vi "arch spiral FGV.vi"(0 "X Start":fxp<+/-,32,16>, 1 "Spiral Step Size":fxp<+/-,32,16>, 2 "Max radius":fxp<+/-,32,16>, 5 "Y Start":fxp<+/-,32,16>, 7 "Action":T1, 9 "Spiral Rotation Direction":T3, 11 "Radial direction":T2=enum."Inward", 12 "Det Frequency":fxp<+,32,0>=0.9999999997671694, 13 "Traj Frequency":fxp<+,32,0>=0.9999999997671694) -> (4 "X position":fxp<+/-,32,16>, 6 "Y position":fxp<+/-,32,16>, 10 "Number of positions":u32, 15 "Trajectory Complete":bool)   [LabVIEW 2015]
uses:
  spiral rotation direction.ctl
  spiral radial direction.ctl
  Trajectory FGV states.ctl
  <vilib>/rvi/FXPMathLib/FxpSinAndCos/subVIs/nifxpmath_SinAndCos_SimConfig.ctl
  <vilib>/rvi/Emulation/niFpgaGetClockAttributes.vi
  <vilib>/rvi/Emulation/niFpgaSctlEmulationGetInTimedLoop.vi
  <vilib>/rvi/Emulation/niFpgaEmulationReportErrorSimple.vi
  <vilib>/rvi/FXPMathLib/FxpSinAndCos/simVIs/DllFxpSinAndCosTemp_sub.vi
  <vilib>/rvi/Emulation/niFpgaCriticalErrorInLSC.vi
  <vilib>/rvi/FXPMathLib/FxpSinAndCos/XNode/nifxpmath_SinAndCos.xnode
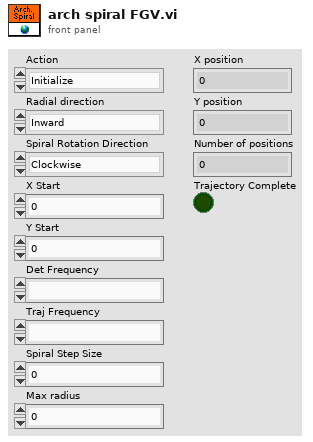
[diagram p1: front panel]
types:
  T1 = typedef "Trajectory FGV states.ctl" = enum16{"Initialize", "Increment"}
  T2 = typedef "spiral radial direction.ctl" = enum16{"Outward", "Inward"}
  T3 = typedef "spiral rotation direction.ctl" = enum16{"Clockwise", "Anti-clockwise"}
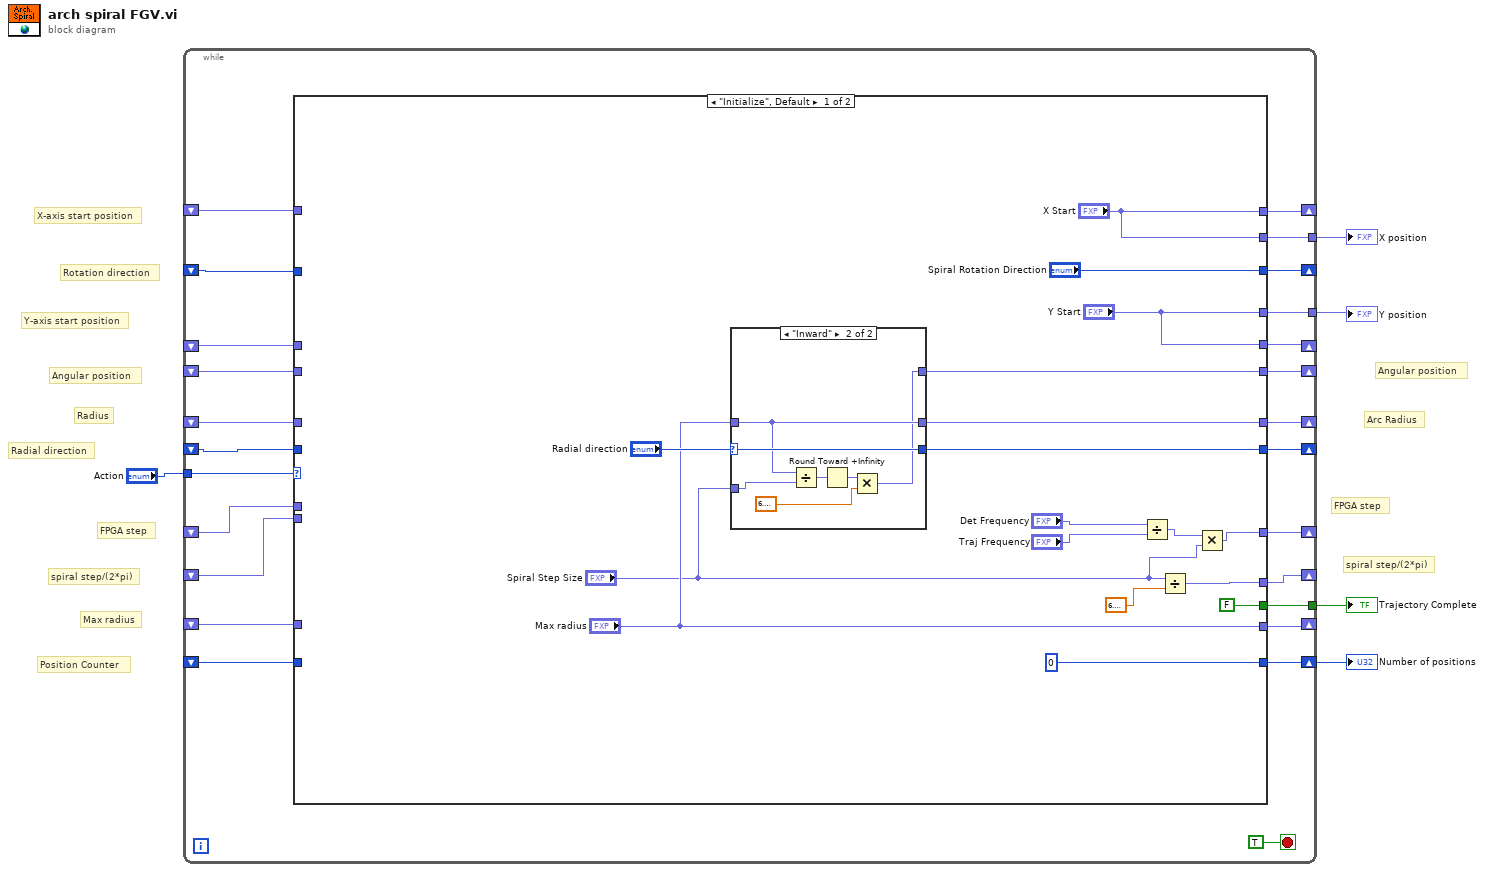
[diagram p0: block diagram]
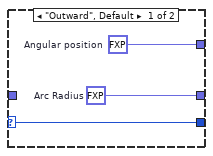
[diagram p2: hidden frame]
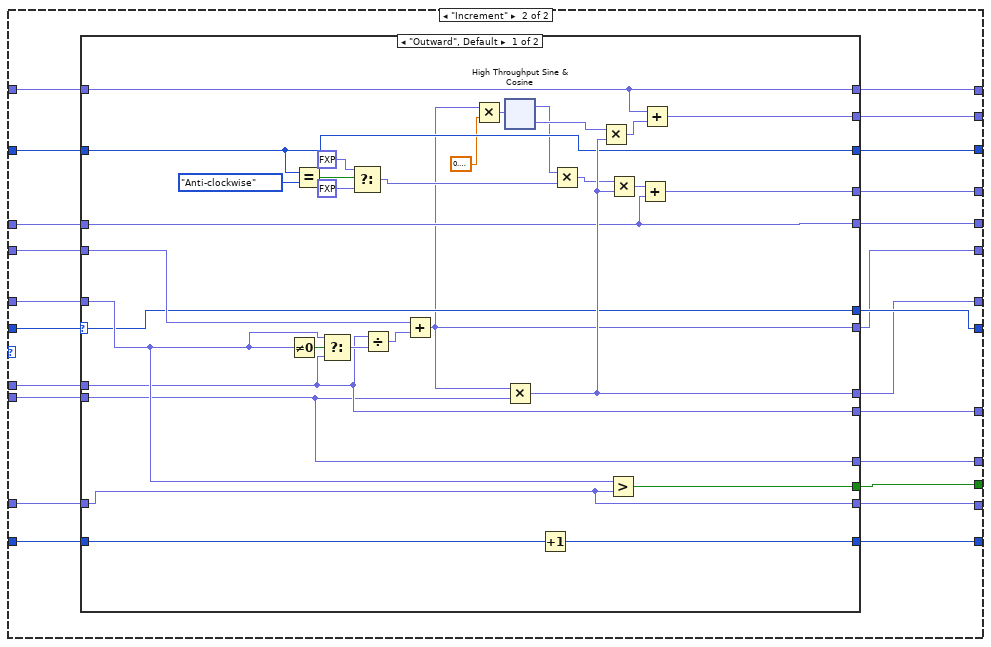
[diagram p3: hidden frame]
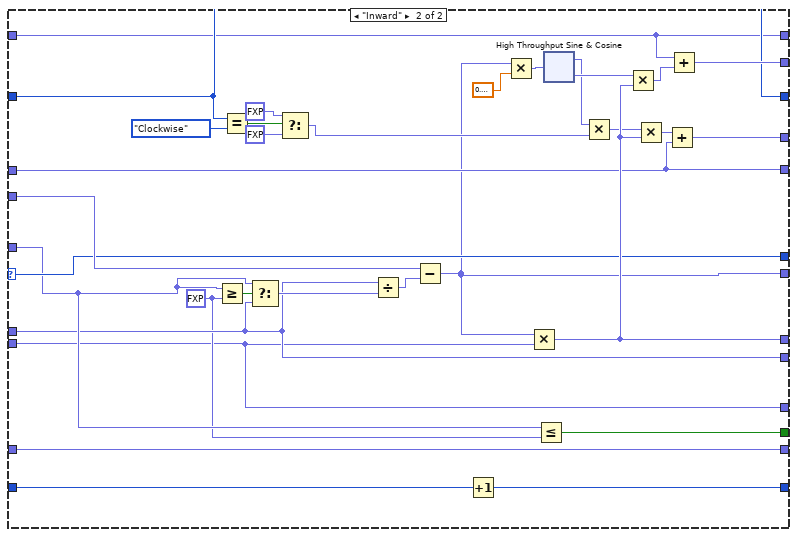
[diagram p4: hidden frame]
diagram:
  # "FPGA step"
  # "spiral step/(2*pi)"
  # "Angular position"
  # "Arc Radius"
  # "Radius"
  # "Angular position"
  # "Radial direction"
  # "Rotation direction"
  # "Position Counter"
  # "X-axis start position"
  # "Y-axis start position"
  # "FPGA step"
  # "spiral step/(2*pi)"
  # "Max radius"
  n1 = while {
    tunnel: "Action" -> [w29]
    shift-right: [w7] -> _
    shift-left: _ -> [w27]
    shift-right: [w6] -> _
    shift-left: _ -> [w28]
    tunnel: [w9] -> w4
    tunnel: [w8] -> w3
    shift-right: [w22] -> _
    shift-left: _ -> [w25]
    shift-right: [w23] -> _
    shift-left: _ -> [w24]
    shift-right: [w21] -> _
    shift-left: _ -> [w10]
    shift-right: [w19] -> _
    shift-left: _ -> [w20]
    shift-right: [w18] -> _
    shift-left: _ -> [w26]
    tunnel: [w17] -> w2
    shift-right: [w16] -> w1
    shift-left: _ -> [w15]
    shift-right: [w14] -> _
    shift-left: _ -> [w13]
    shift-right: [w12] -> _
    shift-left: _ -> [w11]
    stop <- TRUE stop-if-true
    n2 = case shown="\"Initialize\", Default" w29 {
      tunnel: w28 -> [_ w80]
      tunnel: w27 -> [_ w76]
      tunnel: w20 -> [_ w77]
      tunnel: w26 -> [_ w72]
      tunnel: w25 -> [_ w79]
      tunnel: w24 -> [_ w78]
      tunnel: [w44 w65] -> w23
      tunnel: [w43 w60] -> w22
      tunnel: ["Max radius" w66] -> w21
      tunnel: ["X Start" w63] -> w19
      tunnel: ["Y Start" w64] -> w18
      tunnel: [FALSE w75] -> w17
      tunnel: [u32 0 w73] -> w16
      tunnel: w15 -> [_ w74]
      tunnel: ["Spiral Rotation Direction" w68] -> w14
      tunnel: w13 -> [_ w71]
      tunnel: [w38 w69] -> w12
      tunnel: w11 -> [_ w70]
      tunnel: w10 -> [_ w67]
      tunnel: ["X Start" w62] -> w9
      tunnel: ["Y Start" w61] -> w8
      tunnel: [w33 w59] -> w7
      tunnel: [w32 w58] -> w6
      frame "Initialize", Default {
        n3 = case shown="\"Inward\"" "Radial direction" {
          selector: "Radial direction" -> [w49 w57]
          tunnel: [w50 w56] -> w33
          tunnel: [w49 w57] -> w38
          tunnel: "Max radius" -> [_ w56]
          tunnel: [w48 w52] -> w32
          tunnel: "Spiral Step Size" -> [_ w55]
          frame "Outward", Default {
            w48 = fxp<+,24,16> 0.0  # Angular position
            w50 = fxp<+,24,16> 0.0  # Arc Radius
          }
          frame "Inward" {
            n4 = Divide(x=w56, y=w55) -> (x/y=w54:fxp<+/-,64,33>)
            n5 = Round Toward +Infinity(x=w54) -> (ceil(x): smallest int >= x=w53:fxp<+/-,34,34>)
            n6 = Multiply(x=w53, y=sgl 6.2831855) -> (x*y=w52:fxp<+/-,24,16>)
          }
        }
        n7 = Divide(x="Det Frequency", y="Traj Frequency") -> (x/y=w45:fxp<+,40,8>)
        n8 = Divide(x="Spiral Step Size", y=sgl 6.2831855) -> (x/y=w43:fxp<+/-,24,16>)
        n9 = Multiply(x=w45, y="Spiral Step Size") -> (x*y=w44:fxp<+/-,32,16>)
      }
      frame "Increment" {
        n10 = case shown="\"Outward\", Default" w70 {
          selector: w70 -> [w95 w158]
          tunnel: w80 -> [w107 w169]
          tunnel: w79 -> [w89 w150]
          tunnel: w78 -> [w92 w152]
          tunnel: w77 -> [w90 w154]
          tunnel: w76 -> [w106 w153]
          tunnel: [w105 w168] -> w75
          tunnel: w74 -> [w104 w167]
          tunnel: [w103 w166] -> w73
          tunnel: w72 -> [w91 w155]
          tunnel: [w101 w164] -> w59
          tunnel: [w100 w163] -> w62
          tunnel: [w99 w162] -> w61
          tunnel: w71 -> [w94 w157]
          tunnel: [w95 w158] -> w69
          tunnel: [w94 w157] -> w68
          tunnel: w67 -> [w93 w156]
          tunnel: [w93 w156] -> w66
          tunnel: [w92 w152] -> w65
          tunnel: [w91 w155] -> w64
          tunnel: [w90 w154] -> w63
          tunnel: [w89 w150] -> w60
          tunnel: [w81 w143] -> w58
          frame "Outward", Default {
            n11 = Not Equal To 0?(x=w106) -> (x != 0?=w110:bool)
            n12 = Equal?(x=w94, y=spiral_rotation_direction."Anti-clockwise") -> (x = y?=w97:bool)
            n13 = Select(t=w106, s=w110, f=w92) -> (s? t:f=w109:fxp<+/-,33,17>)
            n14 = Select(t=fxp<+,1,1> 1.0, s=w97, f=fxp<+/-,4,4> -1.0) -> (s? t:f=w85:fxp<+/-,4,4>)
            n15 = Divide(x=w92, y=w109) -> (x/y=w108:fxp<+/-,64,33>)
            n16 = Add(x=w107, y=w108) -> (x+y=w81:fxp<+/-,32,16>)
            n17 = Multiply(x=w81, y=sgl 0.31830987) -> (x*y=w82:fxp<+/-,24,16>)
            n18 = xnode "High Throughput Sine & Cosine"("x (pi)"=w82) -> ("sin(x)"=w84:fxp<+/-,16,2>, "cos(x)"=w88:fxp<+/-,16,2>)
            n19 = Multiply(x=w81, y=w89) -> (x*y=w101:fxp<+/-,32,16>)
            n20 = Increment(x=w104) -> (x+1=w103:u32)
            n21 = Multiply(x=w84, y=w85) -> (x*y=w86:fxp<+/-,32,16>)
            n22 = Multiply(x=w88, y=w101) -> (x*y=w111:fxp<+/-,32,16>)
            n23 = Greater?(x=w106, y=w93) -> (0:w105:bool)
            n24 = Multiply(x=w86, y=w101) -> (x*y=w102:fxp<+/-,32,16>)
            n25 = Add(x=w102, y=w91) -> (x+y=w99:fxp<+/-,32,16>)
            n26 = Add(x=w90, y=w111) -> (x+y=w100:fxp<+/-,32,16>)
          }
          frame "Inward" {
            w151 = fxp<+,3,3> 5.0 ("y")
            n27 = Greater Or Equal?(x=w153, y=w151) -> (x >= y?=w172:bool)
            n28 = Equal?(x=w157, y=spiral_rotation_direction."Clockwise") -> (x = y?=w160:bool)
            n29 = Select(t=w153, s=w172, f=w152) -> (s? t:f=w171:fxp<+/-,33,17>)
            n30 = Select(t=fxp<+,1,1> 1.0, s=w160, f=fxp<+/-,4,4> -1.0) -> (s? t:f=w145:fxp<+/-,4,4>)
            n31 = Divide(x=w152, y=w171) -> (x/y=w170:fxp<+/-,32,16>)
            n32 = Subtract(x=w169, y=w170) -> (x-y=w143:fxp<+/-,32,16>)
            n33 = Increment(x=w167) -> (x+1=w166:u32)
            n34 = Multiply(x=w143, y=sgl 0.31830987) -> (x*y=w144:fxp<+/-,24,16>)
            n35 = Multiply(x=w143, y=w150) -> (x*y=w164:fxp<+/-,32,16>)
            n36 = Less Or Equal?(x=w153, y=w151) -> (x <= y?=w168:bool)
            n37 = xnode "High Throughput Sine & Cosine"("x (pi)"=w144) -> ("sin(x)"=w146:fxp<+/-,16,2>, "cos(x)"=w149:fxp<+/-,16,2>)
            n38 = Multiply(x=w146, y=w145) -> (x*y=w147:fxp<+/-,32,16>)
            n39 = Multiply(x=w149, y=w164) -> (x*y=w173:fxp<+/-,48,18>)
            n40 = Multiply(x=w147, y=w164) -> (x*y=w165:fxp<+/-,32,16>)
            n41 = Add(x=w165, y=w155) -> (x+y=w162:fxp<+/-,32,16>)
            n42 = Add(x=w154, y=w173) -> (x+y=w163:fxp<+/-,32,16>)
          }
        }
      }
    }
  }
  "Number of positions" <- w1
  "X position" <- w4
  "Y position" <- w3
  "Trajectory Complete" <- w2
